vi "nominal video create add label.vi"(8 "error in (no error)":errorcluster, 10 "label":string, 11 "staging":i32) -> (0 "error out":errorcluster, 3 "function return":i32)   [LabVIEW 2020, in "client.lvlib"]
doc: "int32_t nominal_video_create_add_label(int32_t staging, const char *label);"
uses:
  client.lvlib
  bin/nominalClient_64.dll
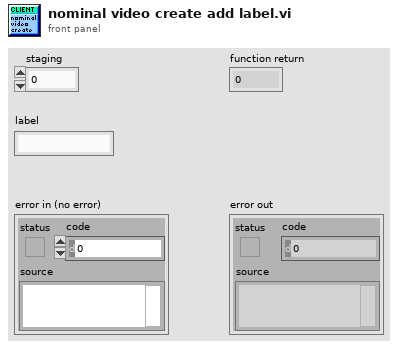
[diagram p1: front panel]
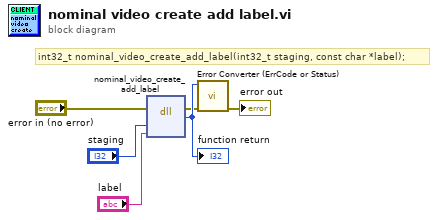
[diagram p0: block diagram]
diagram:
  # "int32_t nominal_video_create_add_label(int32_t staging, const char *label);"
  n1 = dll-call lib="C:/code/labview-client-rs/lv_src/bin/nominalClient_*.*" fn="nominal_video_create_add_label"(error in="error in (no error)", "staging"="staging", "label"="label") -> (error out=w2:errorcluster, w6:i32)  [unwired: 4 in, 1 out]
  "function return" <- w6
  n2 = call "Error Converter (ErrCode or Status).vi"("error in (no error)"=w2, "error code"=w6) -> ("error out"=→"error out":errorcluster)  [unwired: 9 in]
